vi "Test Dequeue Element.vi"() -> ()   [LabVIEW 2013]
uses:
  ByteFIFO/ByteFIFO.lvclass
  VariantBuffer/VariantBuffer.lvclass
panel:
  out "overflow 2":u8[](array[numeric]) format="%02x"
  out "dequeued 2":u8[](array[numeric]) format="%02x"
  out "index2 byte 2":u8 format="%02x"
  out "queue ten elements (array) 2":bool
  out "dequeued elements 2":bool
  out "preview index 2":bool
  out "preview index":bool
  out "dequeued elements":bool
  out "queue ten elements (array)":bool
  out "index2 byte":u8 format="%02x"
  out "dequeued":u8[](array[numeric]) format="%02x"
  out "overflow":u8[](array[numeric]) format="%02x"
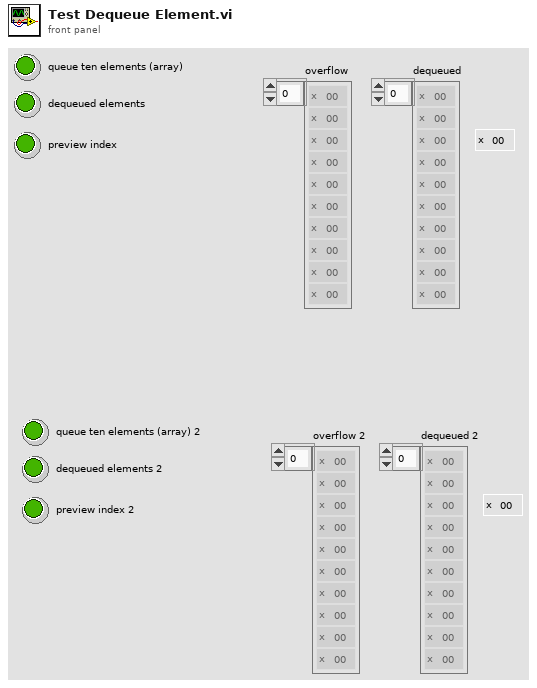
[diagram p1: front panel]
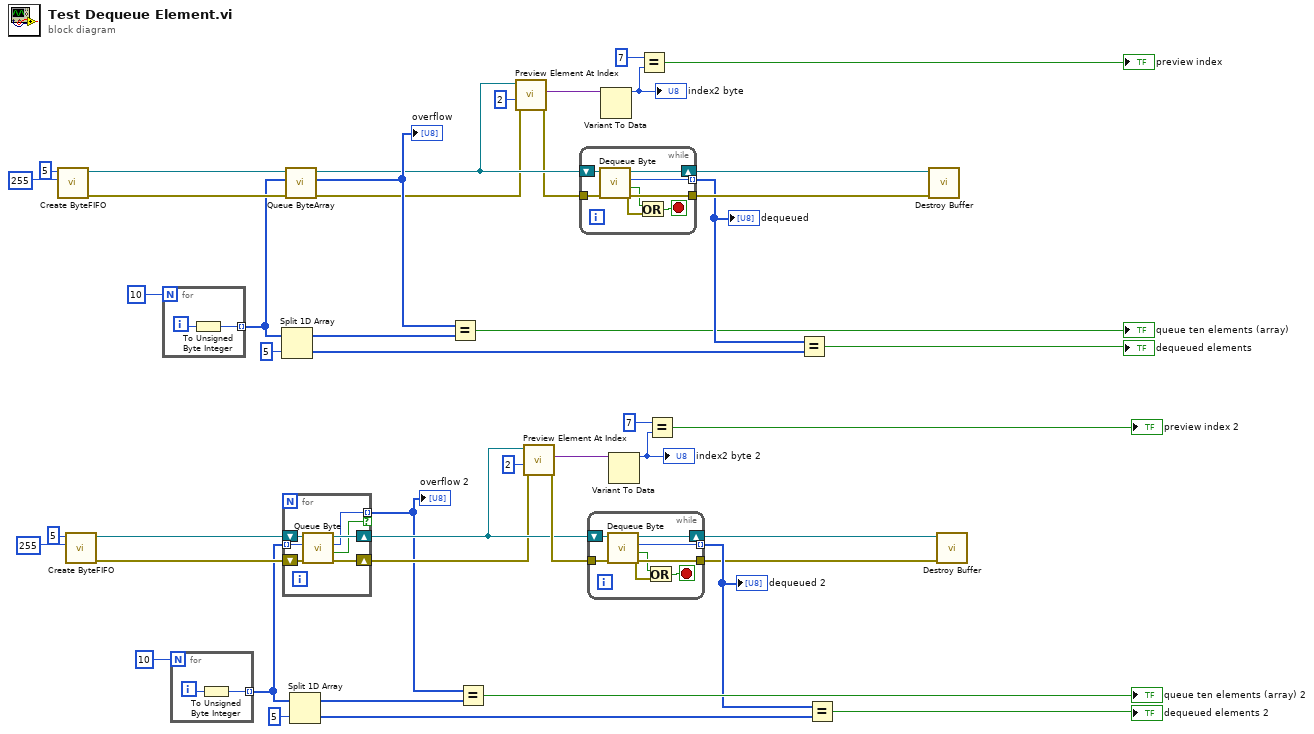
[diagram p0: block diagram]
diagram:
  n1 = call "Create ByteFIFO.vi"("default value"=u8 255, "bufSize"=5) -> ("error out"=w43:errorcluster, "Buffer"=w44:refnum<data-value>)  [unwired: 8 in]
  n2 = call "Create ByteFIFO.vi"("default value"=u8 255, "bufSize"=5) -> ("error out"=w4:errorcluster, "Buffer"=w6:refnum<data-value>)  [unwired: 8 in]
  n3 = for {
    N: 10 -> [_]
    tunnel: [w47] -> w38 mode=indexing
    i -> [w48]
    n4 = To Unsigned Byte Integer(number=w48) -> (unsigned 8bit integer=w47:u8)
  }
  n5 = for {
    N: 10 -> [_]
    tunnel: [w49] -> w2 mode=indexing
    i -> [w50]
    n6 = To Unsigned Byte Integer(number=w50) -> (unsigned 8bit integer=w49:u8)
  }
  n7 = Split 1D Array(array=w38, index=5) -> (first subarray=w36:u8[], second subarray=w35:u8[])
  n8 = for {
    tunnel: w2 -> [w53] mode=indexing
    tunnel: [w52] -> w1 mode=indexing if=w51
    shift-right: [w56] -> w5
    shift-left: w6 -> [w57]
    shift-right: [w54] -> w3
    shift-left: w4 -> [w55]
    n9 = call "Queue Byte.vi"("error in"=w55, "byte"=w53, "Buffer"=w57) -> ("error out"=w54:errorcluster, "overflowed?"=w51:bool, "overflow"=w52:u8, "Buffer"=w56:refnum<data-value>)  [unwired: 5 in]
  }
  "overflow 2" <- w1
  n10 = call "Queue ByteArray.vi"("error in"=w43, "bytes"=w38, "Buffer"=w44) -> ("error out"=w33:errorcluster, "overflow"=w39:u8[], "Buffer"=w34:refnum<data-value>)  [unwired: 6 in]
  "overflow" <- w39
  n11 = Split 1D Array(array=w2, index=5) -> (first subarray=w13:u8[], second subarray=w14:u8[])
  n12 = Equal?(x=w39, y=w36) -> (x = y?=→"queue ten elements (array)":bool)
  n13 = Equal?(x=w1, y=w13) -> (x = y?=→"queue ten elements (array) 2":bool)
  n14 = call "Preview Element At Index.vi"("error in"=w33, "index (-1: last)"=2, "Buffer in"=w34) -> ("error out"=w32:errorcluster, "element"=w30:variant)  [unwired: 5 in, 2 out]
  n15 = call "Preview Element At Index.vi"("error in"=w3, "index (-1: last)"=2, "Buffer in"=w5) -> ("error out"=w15:errorcluster, "element"=w17:variant)  [unwired: 5 in, 2 out]
  n16 = while {
    tunnel: w32 -> [w62]
    tunnel: [w60] -> w40
    tunnel: [w61] -> w27 mode=indexing
    shift-right: [w63] -> w41
    shift-left: w34 -> [w64]
    stop <- w58 stop-if-true
    n17 = call "Dequeue Byte.vi"("error in"=w62, "Buffer"=w64) -> ("error out"=w60:errorcluster, "buffer empty?"=w59:bool, "byte"=w61:u8, "Buffer"=w63:refnum<data-value>)  [unwired: 6 in]
    n18 = Or(x=w59, y=w60) -> (x .or. y?=w58:bool)
  }
  "dequeued" <- w27
  n19 = while {
    tunnel: w15 -> [w69]
    tunnel: [w67] -> w11
    tunnel: [w68] -> w20 mode=indexing
    shift-right: [w70] -> w10
    shift-left: w5 -> [w71]
    stop <- w65 stop-if-true
    n20 = call "Dequeue Byte.vi"("error in"=w69, "Buffer"=w71) -> ("error out"=w67:errorcluster, "buffer empty?"=w66:bool, "byte"=w68:u8, "Buffer"=w70:refnum<data-value>)  [unwired: 6 in]
    n21 = Or(x=w66, y=w67) -> (x .or. y?=w65:bool)
  }
  "dequeued 2" <- w20
  n22 = Variant To Data(Variant=w30) -> (data=w29:u8)  [unwired: 2 in, 1 out]
  "index2 byte" <- w29
  n23 = Variant To Data(Variant=w17) -> (data=w18:u8)  [unwired: 2 in, 1 out]
  "index2 byte 2" <- w18
  n24 = Equal?(x=u8 7, y=w29) -> (x = y?=→"preview index":bool)
  n25 = Equal?(x=u8 7, y=w18) -> (x = y?=→"preview index 2":bool)
  n26 = Equal?(x=w27, y=w35) -> (x = y?=→"dequeued elements":bool)
  n27 = Equal?(x=w20, y=w14) -> (x = y?=→"dequeued elements 2":bool)
  n28 = call "Destroy Buffer.vi"("error in"=w40, "Buffer"=w41) -> ()  [unwired: 8 in, 2 out]
  n29 = call "Destroy Buffer.vi"("error in"=w11, "Buffer"=w10) -> ()  [unwired: 8 in, 2 out]
